vi "Start Timer.vi"(8 "error in (no error)":errorcluster, 10 "Duration":dbl, 11 "Chef Actor in":refnum<class "Chef Actor.lvclass">) -> (0 "error out":errorcluster, 3 "Chef Actor out":refnum<class "Chef Actor.lvclass">)   [LabVIEW 2024, in "Chef Actor.lvlib" / "Chef Actor.lvclass"]
uses:
  Chef Actor.lvclass
  Chef Actor.lvclass/Chef Actor.ctl
  Timer/Timer Messages/Start Counting Msg/Start Counting Msg.lvclass
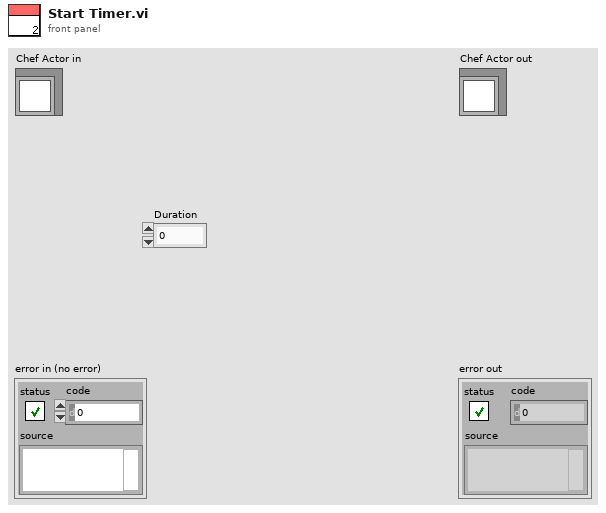
[diagram p1: front panel]
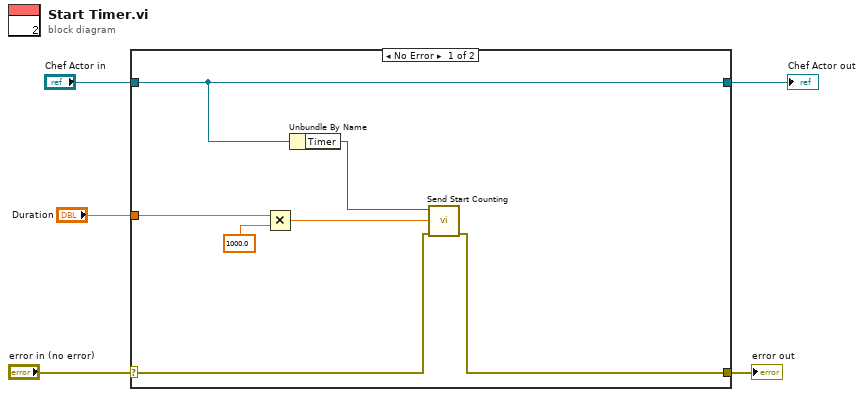
[diagram p0: block diagram]
diagram:
  n1 = case shown="No Error" "error in (no error)" {
    selector: "error in (no error)" -> [w9 w14]
    tunnel: [w8 w14] -> w4
    tunnel: [w12 w13] -> w2
    tunnel: "Chef Actor in" -> [w12 w13]
    tunnel: "Duration" -> [w10 _]
    frame No Error {
      n2 = Multiply(x=w10, y=1000.0) -> (x*y=w7:dbl)
      n3 = Unbundle By Name(w12) -> ("Timer"=w11:refnum<class "Message Enqueuer.lvclass">)
      n4 = call "Send Start Counting.vi"("error in (no error)"=w9, "Duration"=w7, "Message Enqueuer"=w11) -> ("error out"=w8:errorcluster)  [unwired: 7 in, 1 out]
    }
    frame Error {
    }
  }
  "error out" <- w4
  "Chef Actor out" <- w2
